vi "Get Identifier.vi"(8 "error in":errorcluster, 11 "IInstrument in":refnum<class "IInstrument.lvclass">) -> (0 "error out":errorcluster, 2 "Identifier":string, 3 "IInstrument out":refnum<class "IInstrument.lvclass">)   [LabVIEW 2025, in "IInstrument.lvclass"]
uses:
  IInstrument.lvclass
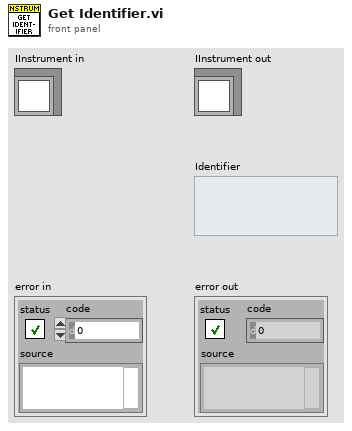
[diagram p1: front panel]
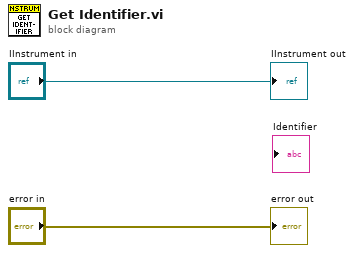
[diagram p0: block diagram]
diagram:
  "error out" <- "error in"
  "IInstrument out" <- "IInstrument in"
